vi "Complete Design.vi"(7 "Result":T1=enum."Valid", 9 "String":string, 11 "Map":T2) -> (3 "Map Out":T2)   [LabVIEW 2024]
uses:
  Map_Track Strings.ctl
  Cluster_Map Data.ctl
  ENUM_String Result.ctl
  Cluster_Parent Data.ctl
  <vilib>/Utility/miscctls.llb/LVMapReplaceAction.ctl
panel:
  out "Current String":string
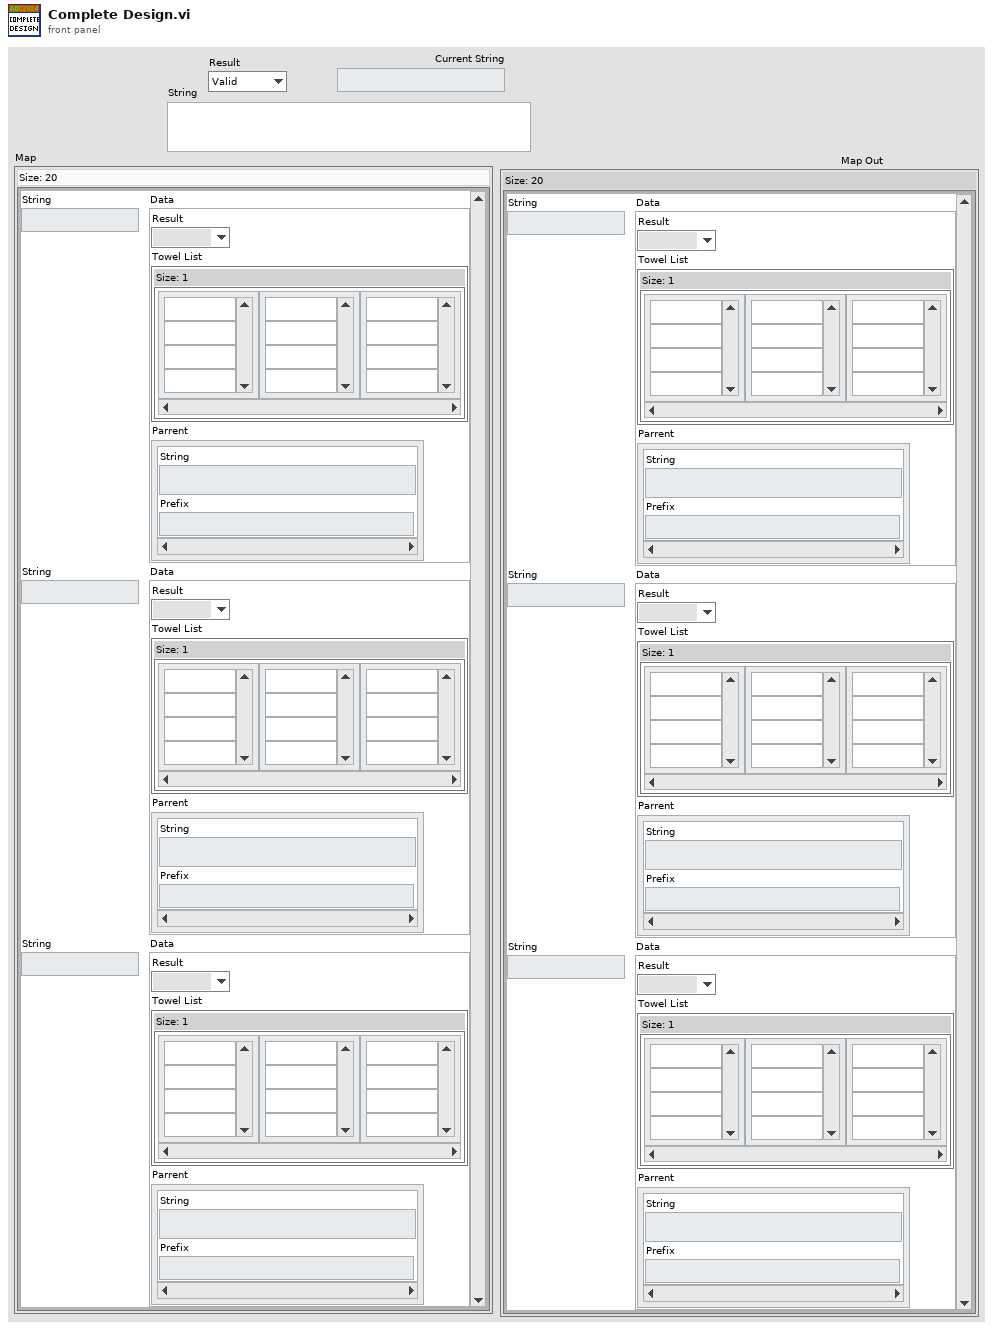
[diagram p1: front panel]
types:
  T1 = typedef "ENUM_String Result.ctl" = enum16{"Unknown", "Invalid", "Valid"}
  T2 = typedef "Map_Track Strings.ctl" = map{string, T3}
  T3 = typedef "Cluster_Map Data.ctl" = cluster{"Result":T1, "Towel List":set{string[]}, "Parrent":T4[]}
  T4 = typedef "Cluster_Parent Data.ctl" = cluster{"String ":string, "Prefix ":string}
  T5 = cluster{"Parrent":T4, "Towel List":set{string[]}}
  T6 = cluster{"Parrent":T4, "Towel List":set{string[]}}[]
  T7 = typedef "LVMapReplaceAction.ctl" = enum32{"Modify Entry only if found", "Add or Modify Entry", "Delete Entry"}
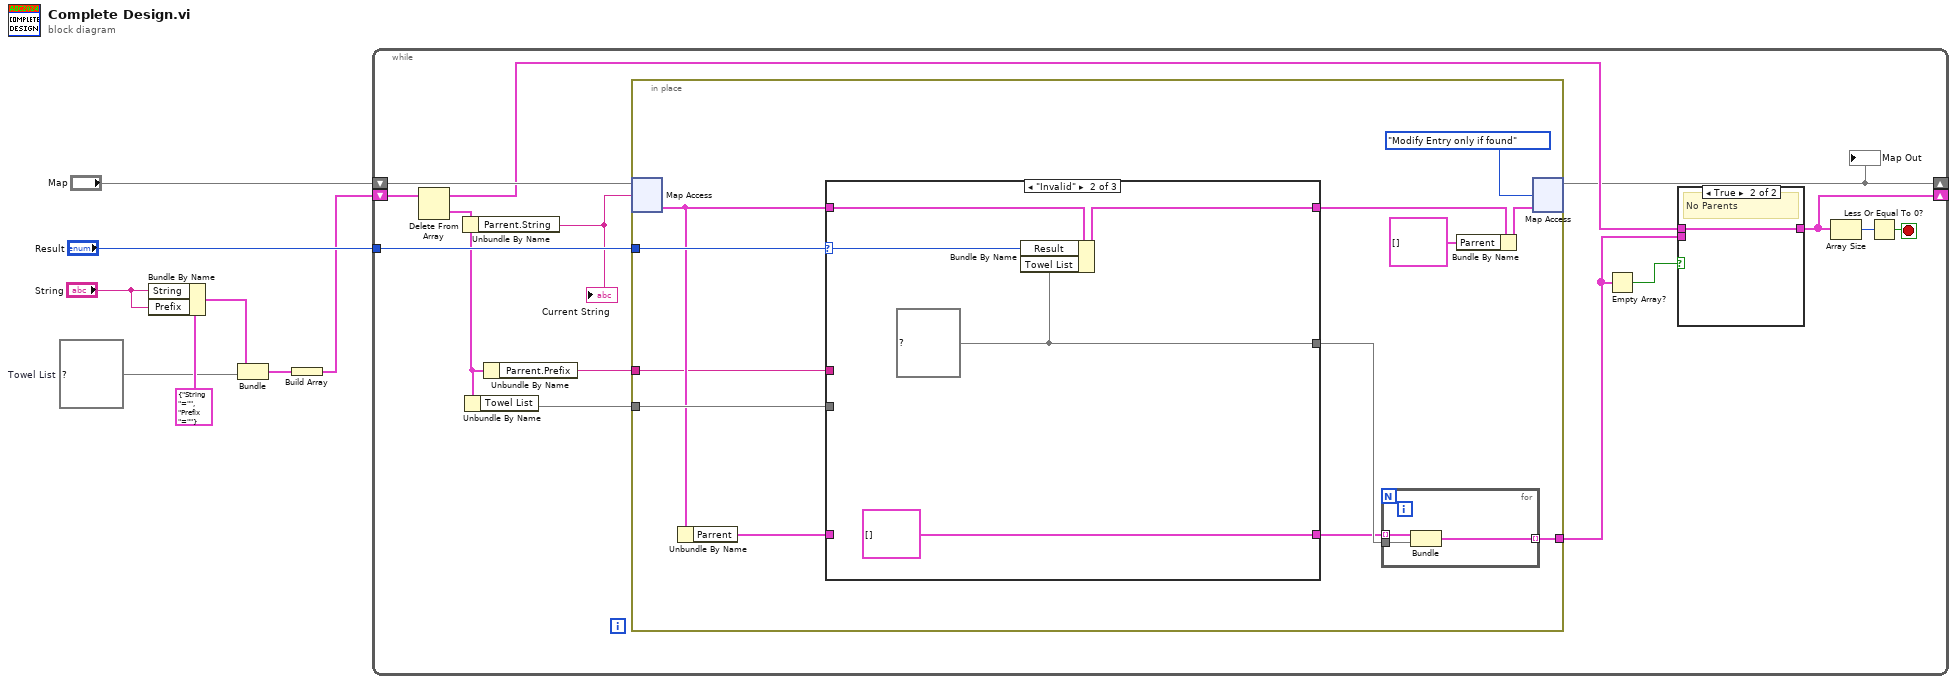
[diagram p0: block diagram]
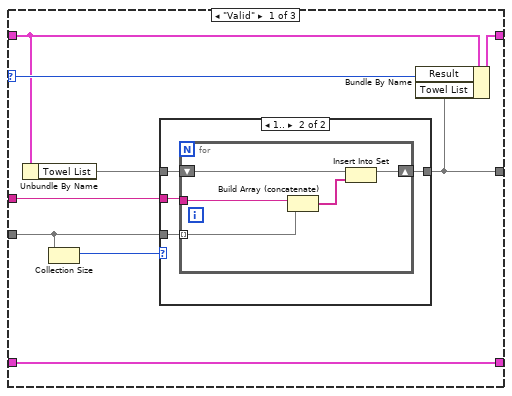
[diagram p2: hidden frame]
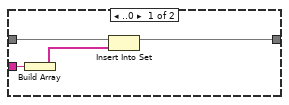
[diagram p3: hidden frame]
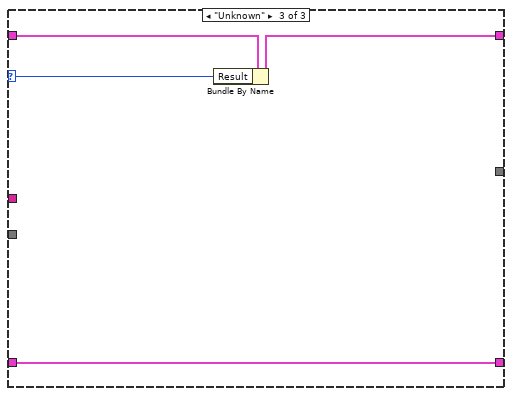
[diagram p4: hidden frame]
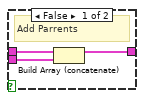
[diagram p5: hidden frame]
diagram:
  w2 = set{string[]} {}  # Towel List
  n1 = Bundle By Name(cluster=T4 {"String "="", "Prefix "=""} ("Parrent"), "String"="String", "Prefix"="String") -> (w4:T4)
  n2 = Bundle("Parrent"=w4, "Towel List"=w2) -> (w6:T5)  [unwired: 1 in]
  n3 = Build Array(w6) -> (w1:T6)
  n4 = while {
    shift-right: [w9] -> _
    shift-left: w1 -> [w10]
    tunnel: "Result" -> [w21]
    shift-right: [w17] -> _
    shift-left: "Map" -> [w22]
    stop <- w18 stop-if-true
    n5 = Delete From Array(array=w10) -> (deleted portion=w12:T5, array with subset deleted=w20:T6)  [unwired: 2 in]
    n6 = Unbundle By Name(w12) -> ("Parrent.String"=w14:string)
    "Current String" <- w14
    n7 = Unbundle By Name(w12) -> ("Towel List"=w13:set{string[]})
    n8 = Unbundle By Name(w12) -> ("Parrent.Prefix"=w11:string)
    n9 = in-place {
      in-place-border: [w28] -> w16
      in-place-border: w13 -> [w33]
      in-place-border: w21 -> [w32]
      in-place-border: w11 -> [w27]
      n10 = in-place-map #1(w22, w14) -> (w31:T3)  [unwired: 1 in, 1 out]
      n11 = Unbundle By Name(w31) -> ("Parrent"=w24:T4[])
      n12 = case shown="\"Invalid\"" w32 {
        selector: w32 -> [w42 w60 w64]
        tunnel: [w43 w61 w65] -> w30
        tunnel: w33 -> [w37 _ _]
        tunnel: [w38 w58 _] -> w25
        tunnel: w31 -> [w40 w59 w63]
        tunnel: w27 -> [w41 _ _]
        tunnel: w24 -> [w35 _ w62]
        tunnel: [w35 T4[] [] ("Parrent") w62] -> w23
        frame "Valid" {
          n13 = Unbundle By Name(w40) -> ("Towel List"=w39:set{string[]})
          n14 = Collection Size(1:w37) -> (0:w36:i32)
          n15 = case shown="1.." w36 {
            tunnel: w37 -> [_ w51]
            tunnel: w41 -> [w47 w50]
            tunnel: w39 -> [w46 w49]
            tunnel: [w45 w48] -> w38
            frame ..0 {
              n16 = Build Array(w47) -> (w44:string[])
              n17 = Insert Into Set(10:w44, 11:w46) -> (3:w45:set{string[]})  [unwired: 1 out]
            }
            frame 1.. {
              n18 = for {
                tunnel: w51 -> [w52] mode=indexing
                tunnel: w50 -> [w56]
                shift-right: [w53] -> w48
                shift-left: w49 -> [w55]
                n19 = Build Array (concatenate)(w56, w52) -> (w54:string[])
                n20 = Insert Into Set(10:w54, 11:w55) -> (3:w53:set{string[]})  [unwired: 1 out]
              }
            }
          }
          n21 = Bundle By Name(cluster=w40, "Result"=w42, "Towel List"=w38) -> (w43:T3)
        }
        frame "Invalid" {
          w58 = set{string[]} {} ("Towel List")
          n22 = Bundle By Name(cluster=w59, "Result"=w60, "Towel List"=w58) -> (w61:T3)
        }
        frame "Unknown" {
          n23 = Bundle By Name(cluster=w63, "Result"=w64) -> (w65:T3)
        }
      }
      n24 = for {
        tunnel: w23 -> [w68] mode=indexing
        tunnel: [w67] -> w28 mode=indexing
        tunnel: w25 -> [w66]
        n25 = Bundle("Parrent"=w68, "Towel List"=w66) -> (w67:T5)  [unwired: 1 in]
      }
      n26 = Bundle By Name(cluster=w30, "Parrent"=T4[] []) -> (w29:T3)
      n27 = in-place-map #1(w29, LVMapReplaceAction."Modify Entry only if found" ("action")) -> (w17:T2)  [unwired: 2 out]
    }
    "Map Out" <- w17
    n28 = Empty Array?(array=w16) -> (empty?=w15:bool)
    n29 = case shown="True" w15 {
      tunnel: w20 -> [w71 w72]
      tunnel: [w70 w72] -> w9
      tunnel: w16 -> [w69 _]
      frame False {
        # "Add Parrents"
        n30 = Build Array (concatenate)(w71, w69) -> (w70:T6)
      }
      frame True {
        # "No Parents"
      }
    }
    n31 = Array Size(array=w9) -> (size(s)=w19:i32)
    n32 = Less Or Equal To 0?(x=w19) -> (x <= 0?=w18:bool)
  }
